vi "Write byte order.vi"(8 "error in (no error)":errorcluster, 10 "byte order":T1(ring), 11 "Configuration.Transfer in":refnum<class "Configuration.Transfer.lvclass">) -> (0 "error out":errorcluster, 3 "Configuration.Transfer out":refnum<class "Configuration.Transfer.lvclass">)   [LabVIEW 2016, in "Data Sharing Framework.Configuration.lvlib" / "Configuration.Transfer.lvclass"]
uses:
  Configuration.Transfer.lvclass
  Configuration.Transfer.lvclass/Configuration.Transfer.ctl
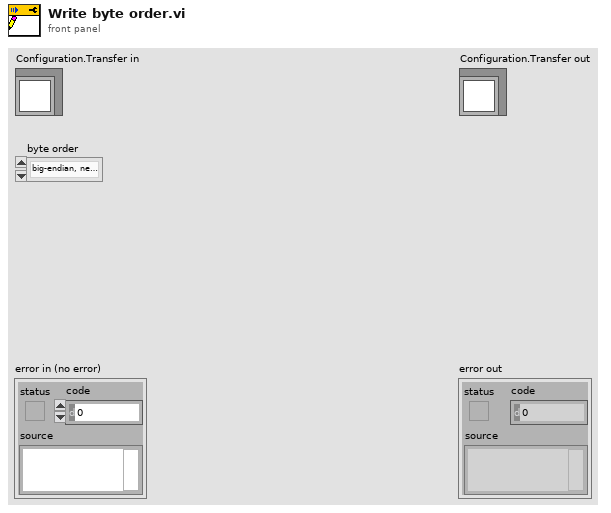
[diagram p1: front panel]
types:
  T1 = enum16{"big-endian, network order", "native, host order", "little-endian"}
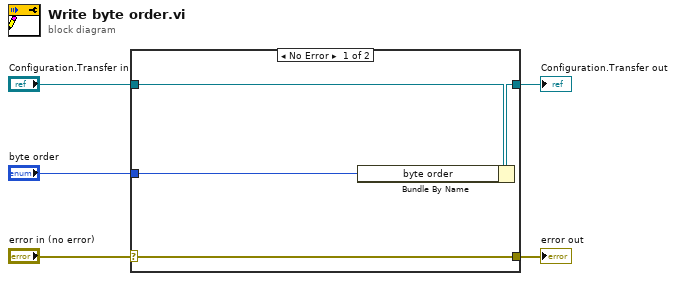
[diagram p0: block diagram]
diagram:
  n1 = case shown="No Error" "error in (no error)" {
    selector: "error in (no error)" -> [w9 w10]
    tunnel: [w9 w10] -> w4
    tunnel: [w7 w11] -> w2
    tunnel: "Configuration.Transfer in" -> [w8 w11]
    tunnel: "byte order" -> [w6 _]
    frame No Error {
      n2 = Bundle By Name(cluster=w8, "byte order"=w6) -> (w7:refnum<class "Configuration.Transfer.lvclass">)
    }
    frame Error {
    }
  }
  "error out" <- w4
  "Configuration.Transfer out" <- w2
